vi "read.vi"(8 "error in (no error)":errorcluster, 10 "ILC":refnum<class "ILC.lvclass">, 11 "ReadILCLIMSW1Strategy in":refnum<class "ReadILCLIMSW2Strategy.lvclass">) -> (0 "error out":errorcluster, 2 "Value":dbl, 3 "ReadILCLIMSW1Strategy out":refnum<class "ReadILCLIMSW2Strategy.lvclass">)   [LabVIEW 2015, in "ReadILCLIMSW2Strategy.lvclass"]
uses:
  ReadILCLIMSW2Strategy.lvclass
  <userlib>/Common/ILC/ILC/ILC.lvclass
  <userlib>/Common/ILC/ILC/ILC.lvclass/ILC.ctl
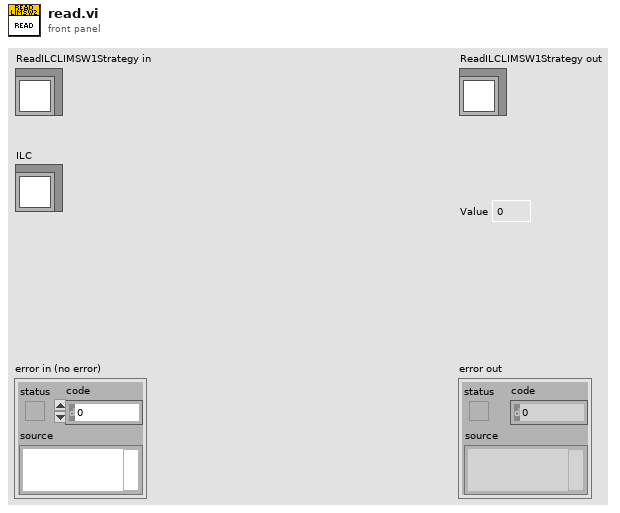
[diagram p1: front panel]
types:
  T1 = typedef "ILCCommon.lvlib/ILCTypedefs.lvlib/InputData.ctl" = cluster{"Input Channels":T2, "Limit Switches":T3, "Tachometer":u16, "SSI Encoder":i32, "ADCs":T4}
  T2 = typedef "ILCCommon.lvlib/ILCConfiguration.lvlib/InputChannels.ctl" = enum16{"Channel 0", "3 Channels", "5 Channels"}
  T3 = typedef "ILCCommon.lvlib/ILCTypedefs.lvlib/LimitSwitches.ctl" = cluster{"1":bool, "2":bool}
  T4 = typedef "ILCCommon.lvlib/ILCTypedefs.lvlib/ADCs.ctl" = cluster{"Ch0":i32, "Ch1":i32, "Ch2":i32, "Ch3":i32, "Ch4":i32}
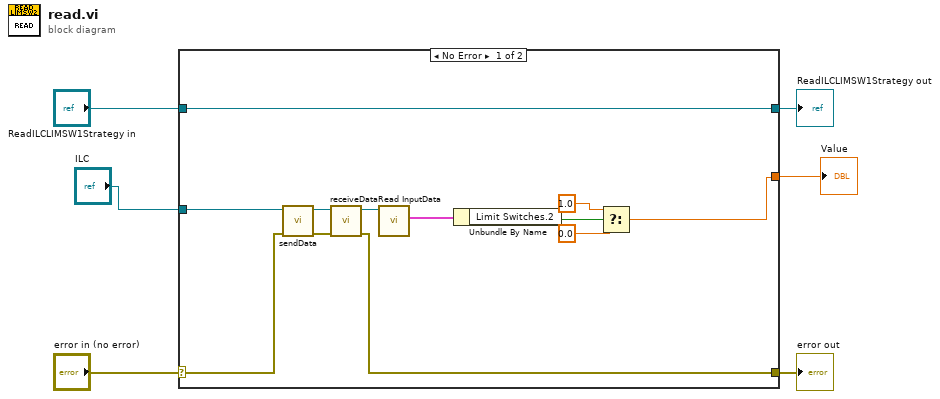
[diagram p0: block diagram]
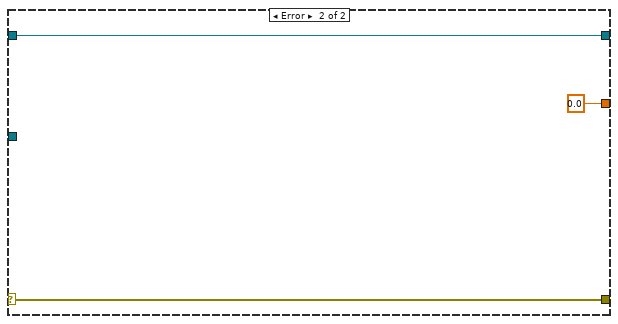
[diagram p2: hidden frame]
diagram:
  n1 = case shown="No Error" "error in (no error)" {
    selector: "error in (no error)" -> [w13 w21]
    tunnel: [w11 w21] -> w5
    tunnel: [w18 w20] -> w3
    tunnel: "ReadILCLIMSW1Strategy in" -> [w18 w20]
    tunnel: [w7 0.0 ("Value")] -> w2
    tunnel: "ILC" -> [w17 _]
    frame No Error {
      n2 = call <userlib>:"sendData.vi"("error in (no error)"=w13, "ILC in"=w17) -> ("error out"=w12:errorcluster, "ILC out"=w16:refnum<class "ILC.lvclass">)  [unwired: 8 in]
      n3 = call <userlib>:"receiveData.vi"("error in (no error)"=w12, "ILC in"=w16) -> ("error out"=w11:errorcluster, "ILC out"=w15:refnum<class "ILC.lvclass">)  [unwired: 8 in]
      n4 = call <userlib>:"Read InputData.vi"("ILC in"=w15) -> ("InputData"=w14:T1)  [unwired: 9 in, 1 out]
      n5 = Unbundle By Name(w14) -> ("Limit Switches.2"=w10:bool)
      n6 = Select(t=1.0, s=w10, f=0.0) -> (s? t:f=w7:dbl)
    }
    frame Error {
    }
  }
  "error out" <- w5
  "ReadILCLIMSW1Strategy out" <- w3
  "Value" <- w2
